vi "Comments.Add Wiring Description.vi"(8 "error in (no error)":errorcluster, 11 "Control Experiment in":refnum<class "Control Experiment.lvclass">) -> (0 "error out":errorcluster, 3 "Control Experiment out":refnum<class "Control Experiment.lvclass">)   [LabVIEW 2016, in "Control Experiment.lvclass"]
uses:
  Control Experiment.lvclass
  Control Experiment.lvclass/Control Experiment.ctl
  <userlib>/LevyLab/Krohn Hite 7008/Instrument.KH7008.lvclass/Instrument.KH7008.ctl
  <userlib>/LevyLab/Krohn Hite 7008/Instrument.KH7008.lvclass
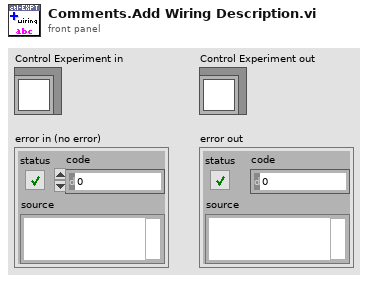
[diagram p1: front panel]
types:
  T1 = typedef "Instrument.KH7008.lvclass/KH_control_array.ctl" = T2[]
  T2 = typedef "Instrument.KH7008.lvclass/KH_control.ctl" = cluster{"Channel":T3, "Gain":T4, "Shunt Resistor":T5, "Input Config":T6}
  T3 = typedef "Instrument.KH7008.lvclass/Channel-Enum.ctl" = enum16{"Channel 1", "Channel 2", "Channel 3", "Channel 4", "Channel 5", "Channel 6", "Channel 7", "Channel 8"}
  T4 = typedef "Instrument.KH7008.lvclass/Gain-Enum.ctl" = enum16{"1x", "10x", "100x", "1000x"}
  T5 = typedef "Instrument.KH7008.lvclass/Shunt-Enum.ctl" = enum16{"Open", "50 Ohms", "500 Ohms", "5k Ohms", "50k Ohms"}
  T6 = typedef "Instrument.KH7008.lvclass/Input Configuration-Enum.ctl" = enum16{"Ground", "SE+ (-gnd)", "SE- (+gnd)", "Differential"}
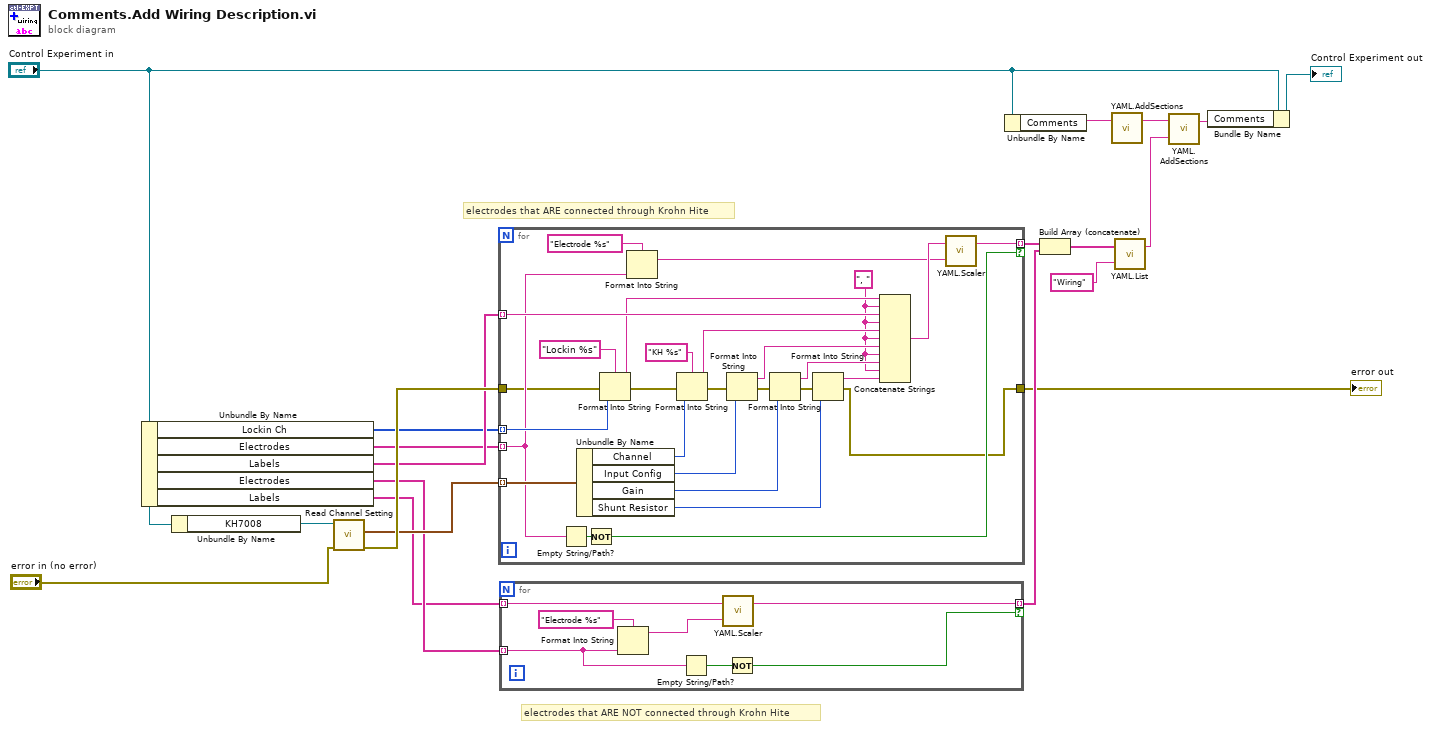
[diagram p0: block diagram]
diagram:
  # "electrodes that ARE NOT connected through Krohn Hite"
  # "electrodes that ARE connected through Krohn Hite"
  n1 = Unbundle By Name("Control Experiment in") -> ("Lockin Ch"=w5:enum16{"1", "2", "3", "4", "5", "6", "7", "8"}[], "Electrodes"=w6:string[], "Labels"=w10:string[], "Electrodes"=w8:string[], "Labels"=w7:string[])
  n2 = Unbundle By Name("Control Experiment in") -> ("KH7008"=w9:refnum<class "Instrument.KH7008.lvclass">)
  n3 = call <userlib>:"Read Channel Setting.vi"("error in (no error)"="error in (no error)", "Instrument.KH7008 in"=w9) -> ("error out"=w12:errorcluster, "Channel Setting"=w11:T1)  [unwired: 7 in, 1 out]
  n4 = for {
    tunnel: w5 -> [w43] mode=indexing
    tunnel: w6 -> [w32] mode=indexing
    tunnel: w10 -> [w44] mode=indexing
    tunnel: [w22] -> w14 mode=indexing if=w39
    tunnel: w12 -> [w31]
    tunnel: [w25] -> w4
    tunnel: w11 -> [w38] mode=indexing
    w21 = ", "
    n5 = Empty String/Path?(string/path=w32) -> (empty?=w40:bool)
    n6 = Unbundle By Name(w38) -> ("Channel"=w37:T3, "Input Config"=w36:T6, "Gain"=w35:T4, "Shunt Resistor"=w34:T5)
    n7 = Not(x=w40) -> (.not. x?=w39:bool)
    n8 = Format Into String(format string="Lockin %s", error in=w31, w43) -> (resulting string=w27:string, error out=w42:errorcluster)  [unwired: 1 in]
    n9 = Format Into String(format string="Electrode %s", w32) -> (resulting string=w23:string)  [unwired: 2 in, 1 out]
    n10 = Format Into String(format string="KH %s", error in=w42, w37) -> (resulting string=w28:string, error out=w47:errorcluster)  [unwired: 1 in]
    n11 = Format Into String(error in=w47, w36) -> (resulting string=w26:string, error out=w46:errorcluster)  [unwired: 2 in]
    n12 = Format Into String(error in=w46, w35) -> (resulting string=w41:string, error out=w45:errorcluster)  [unwired: 2 in]
    n13 = Format Into String(error in=w45, w34) -> (resulting string=w48:string, error out=w25:errorcluster)  [unwired: 2 in]
    n14 = Concatenate Strings(w27, w21, w44, w21, w28, w21, w26, w21, w41, w21, w48) -> (w24:string)
    n15 = call "YAML.Scaler.vi"("Key"=w23, "Scaler"=w24) -> ("Output"=w22:string)  [unwired: 1 in]
  }
  "error out" <- w4
  n16 = for {
    tunnel: [w49] -> w15 mode=indexing if=w53
    tunnel: w7 -> [w50] mode=indexing
    tunnel: w8 -> [w55] mode=indexing
    n17 = Format Into String(format string="Electrode %s", w55) -> (resulting string=w51:string)  [unwired: 2 in, 1 out]
    n18 = Empty String/Path?(string/path=w55) -> (empty?=w54:bool)
    n19 = call "YAML.Scaler.vi"("Key"=w51, "Scaler"=w50) -> ("Output"=w49:string)  [unwired: 1 in]
    n20 = Not(x=w54) -> (.not. x?=w53:bool)
  }
  n21 = Unbundle By Name("Control Experiment in") -> ("Comments"=w17:string)
  n22 = Build Array (concatenate)(w14, w15) -> (w16:string[])
  n23 = call "YAML.AddSections.vi"("Section 1"=w17) -> ("Output"=w19:string)  [unwired: 2 in]
  n24 = call "YAML.List.vi"("Key"="Wiring" ("string"), "lines"=w16) -> ("Output"=w1:string)  [unwired: 1 in]
  n25 = call "YAML.AddSections.vi"("Section 2"=w1, "Section 1"=w19) -> ("Output"=w20:string)  [unwired: 1 in]
  n26 = Bundle By Name(cluster="Control Experiment in", "Comments"=w20) -> (→"Control Experiment out":refnum<class "Control Experiment.lvclass">)
